vi "User-Defined IO Variable - Basic-PXI.vi"   [LabVIEW 2015]
uses:
  <vilib>/rvi/Emulation/niFpgaGetClockAttributes.vi
  <vilib>/rvi/Emulation/niFpgaSctlEmulationGetInTimedLoop.vi
  <vilib>/rvi/Emulation/niFpgaEmulationReportErrorSimple.vi
  <vilib>/rvi/eio/common/nirviEmuTemplateMethod_errors.vi
  <vilib>/rvi/Emulation/niFpgaCriticalErrorInLSC.vi
  <vilib>/eio/EIONode/EIONode.xnode
panel:
  # "See block diagram"
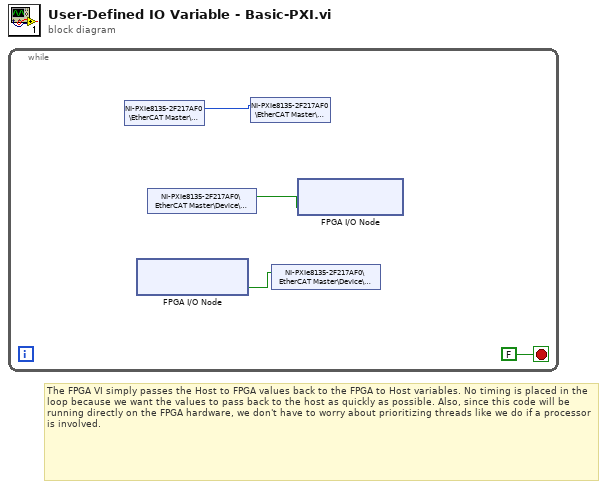
[diagram p0: block diagram]
diagram:
  # "The FPGA VI simply passes the Host to FPGA values back to the FPGA to Host variables. No timing is placed in the loop because we want the values to pass back to the host as quickly as possible. Also, since this code will be running directly on the FPGA hardware, we don't have to worry about prioritizing threads like we do if a processor is involved."
  n1 = while {
    stop <- FALSE stop-if-true
    n2 = shared-variable "NI-PXIe8135-2F217AF0\\EtherCAT Master\\Device\\User-Defined Variables\\HF: Int"() -> (w1:u32)  [unwired: 1 in, 1 out]
    n3 = xnode "FPGA I/O Node"() -> ("Mod8/DIO16"=w3:bool)  [unwired: 1 in, 1 out]
    n4 = shared-variable "NI-PXIe8135-2F217AF0\\EtherCAT Master\\Device\\User-Defined Variables\\HF: Boolean"() -> (w2:bool)  [unwired: 1 in, 1 out]
    n5 = shared-variable "NI-PXIe8135-2F217AF0\\EtherCAT Master\\Device\\User-Defined Variables\\FH: Int"(w1) -> ()  [unwired: 1 in, 1 out]
    n6 = shared-variable "NI-PXIe8135-2F217AF0\\EtherCAT Master\\Device\\User-Defined Variables\\FH: Boolean"(w3) -> ()  [unwired: 1 in, 1 out]
    n7 = xnode "FPGA I/O Node"("Mod8/DIO0"=w2) -> ()  [unwired: 1 in, 1 out]
  }
